vi "Check AI3 BAE7.vi"(0 "error in":errorcluster) -> (14 "error out":errorcluster, 16 "voltage out":dbl format="%#_13g")   [LabVIEW 2014]
doc: "Check AI3 BAE7\n\nThis returns the voltage inputted into AI3, which serves as the analog input receiving ~ 5 V through DC.\n\nBeverly Abadines\nPHY 350\nE7"
uses:
  <vilib>/DAQmx/read.llb/DAQmx Read.vi
  <vilib>/DAQmx/read.llb/DAQmx Read (Analog 1D DBL NChan 1Samp).vi
  <vilib>/DAQmx/miscellaneous.llb/DAQmx Fill In Error Info.vi
  <vilib>/DAQmx/create/channels.llb/DAQmx Create Channel (AI-Voltage-Basic).vi
  <vilib>/DAQmx/create/channels.llb/DAQmx Create Channel (TEDS-AI-Voltage-Basic).vi
panel:
  out "device out":tag="Dev1"
  in  "device in":tag="Dev1"
  in  "stop (T)":bool=TRUE
  in  "timeout (s)":dbl=10.0 format="%0.2f"
  out "task out":refnum<k21>
  # "Check AI3 BAE7"
  # "Beverly Abadines\nPhys 350\nE7"
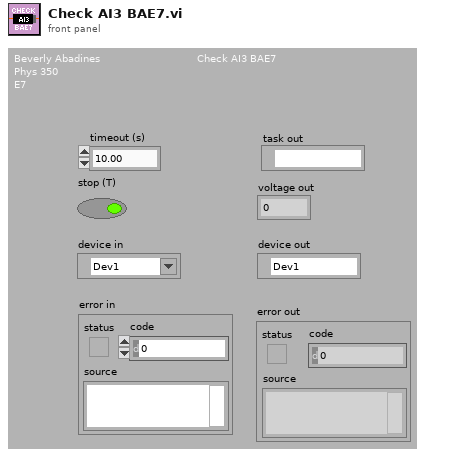
[diagram p1: front panel]
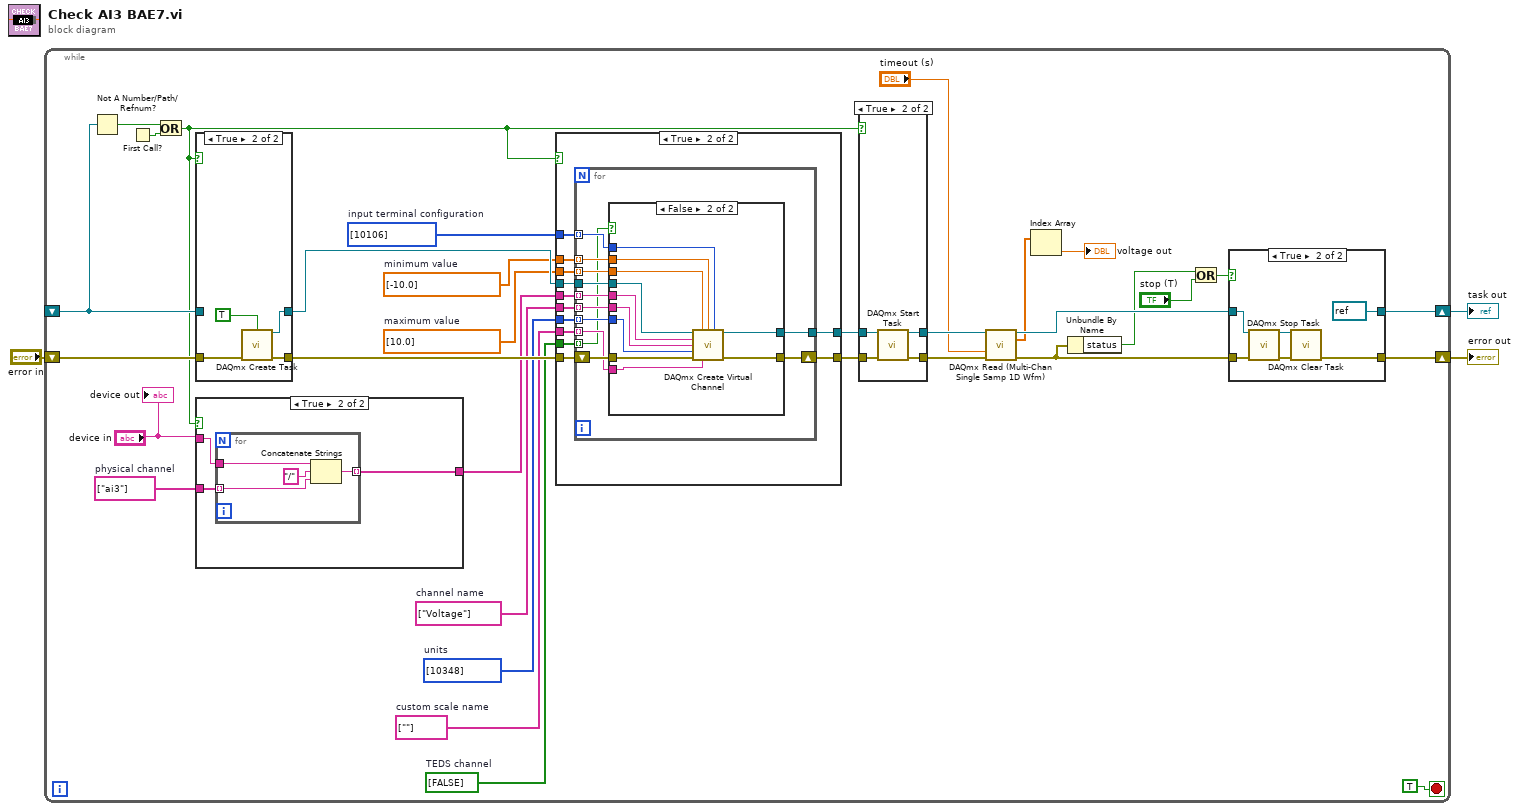
[diagram p0: block diagram]
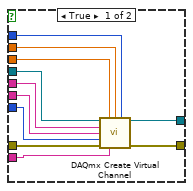
[diagram p5: hidden frame]
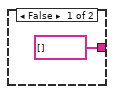
[diagram p6: hidden frame]
diagram:
  n1 = while {
    shift-right: [w12] -> w1
    shift-left: _ -> [w32]
    shift-right: [w10] -> w2
    shift-left: "error in" -> [w33]
    stop <- TRUE stop-if-true
    w19 = bool[] [FALSE]  # TEDS channel
    w20 = string[] [""]  # custom scale name
    w21 = i32[] [10348] items=["Volts"=10348, "From TEDS"=12516, "From Custom Scale"=10065]  # units
    w22 = string[] ["Voltage"]  # channel name
    w24 = dbl[] [10.0]  # maximum value
    w25 = dbl[] [-10.0]  # minimum value
    w26 = i32[] [10106] items=["default"=-1, "RSE"=10083, "NRSE"=10078, "Differential"=10106, "Pseudodifferential"=12529]  # input terminal configuration
    w29 = string[] ["ai3"]  # physical channel
    n2 = Not A Number/Path/Refnum?(number/path/refnum=w32) -> (NaN/Path/Refnum?=w31:bool)
    n3 = First Call?() -> (First Call?: T/F=w34:bool)
    n4 = Or(x=w31, y=w34) -> (x .or. y?=w18:bool)
    n5 = case shown="True" w18 {
      tunnel: [w107 w111] -> w28
      tunnel: w32 -> [w107 _]
      tunnel: [w106 w110] -> w27
      tunnel: w33 -> [w106 w108]
      frame False {
      }
      frame True {
        n6 = call <vilib>:"DAQmx Create Task.vi"("auto cleanup"=TRUE, "error in"=w108) -> ("task out"=w111:refnum<k21>, "error out"=w110:errorcluster)  [unwired: 12 in]
      }
    }
    n7 = case shown="True" w18 {
      tunnel: [string[] [] w101] -> w23
      tunnel: "device in" -> [_ w100]
      tunnel: w29 -> [_ w99]
      frame False {
      }
      frame True {
        n8 = for {
          tunnel: [w105] -> w101 mode=indexing
          tunnel: w100 -> [w104]
          tunnel: w99 -> [w102] mode=indexing
          n9 = Concatenate Strings(w104, "/" ("string"), w102) -> (w105:string)
        }
      }
    }
    n10 = case shown="True" w18 {
      tunnel: [w51 w61] -> w17
      tunnel: w28 -> [w51 w63]
      tunnel: [w50 w60] -> w16
      tunnel: w27 -> [w50 w62]
      tunnel: w26 -> [_ w59]
      tunnel: w25 -> [_ w58]
      tunnel: w24 -> [_ w57]
      tunnel: w23 -> [_ w56]
      tunnel: w22 -> [_ w55]
      tunnel: w21 -> [_ w54]
      tunnel: w20 -> [_ w53]
      tunnel: w19 -> [_ w52]
      frame False {
      }
      frame True {
        n11 = for {
          tunnel: w63 -> [w75]
          tunnel: [w73] -> w61
          tunnel: w59 -> [w71] mode=indexing
          tunnel: w58 -> [w70] mode=indexing
          tunnel: w57 -> [w69] mode=indexing
          tunnel: w56 -> [w68] mode=indexing
          tunnel: w55 -> [w67] mode=indexing
          tunnel: w54 -> [w66] mode=indexing
          tunnel: w53 -> [w65] mode=indexing
          shift-right: [w72] -> w60
          shift-left: w62 -> [w74]
          tunnel: w52 -> [w64] mode=indexing
          n12 = case shown="False" w64 {
            tunnel: w75 -> [w86 w97]
            tunnel: w74 -> [w85 w96]
            tunnel: [w84 w95] -> w73
            tunnel: [w83 w94] -> w72
            tunnel: w71 -> [w82 w93]
            tunnel: w70 -> [w81 w92]
            tunnel: w69 -> [w80 w91]
            tunnel: w68 -> [w79 w90]
            tunnel: w67 -> [w78 w89]
            tunnel: w66 -> [w77 w88]
            tunnel: w65 -> [w76 w87]
            frame True {
              n13 = call-poly <vilib>:"DAQmx Create Virtual Channel.vi"("task in"=w86, "maximum value"=w80, "minimum value"=w81, "input terminal configuration"=w82, "physical channels"=w79, "name to assign"=w78, "units"=w77, "error in"=w85, "custom scale name"=w76) -> ("task out"=w84:refnum<k21>, "error out"=w83:errorcluster)  [unwired: 5 in]
            }
            frame False {
              n14 = call-poly <vilib>:"DAQmx Create Virtual Channel.vi"("task in"=w97, "maximum value"=w91, "minimum value"=w92, "input terminal configuration"=w93, "physical channels"=w90, "name to assign"=w89, "units"=w88, "error in"=w96, "custom scale name"=w87) -> ("task out"=w95:refnum<k21>, "error out"=w94:errorcluster)  [unwired: 5 in]
            }
          }
        }
      }
    }
    n15 = case shown="True" w18 {
      tunnel: [w45 w48] -> w15
      tunnel: w17 -> [w45 w49]
      tunnel: [w44 w46] -> w14
      tunnel: w16 -> [w44 w47]
      frame False {
      }
      frame True {
        n16 = call <vilib>:"DAQmx Start Task.vi"("task/channels in"=w49, "error in"=w47) -> ("task out"=w48:refnum<k21>, "error out"=w46:errorcluster)  [unwired: 12 in]
      }
    }
    n17 = call-poly "DAQmx Read (Multi-Chan Single Samp 1D Wfm).vi"("task/channels in"=w15, "timeout"="timeout (s)", "error in"=w14) -> ("task out"=w11:refnum<k21>, "data"=w4:dbl[], "error out"=w9:errorcluster)  [unwired: 10 in]
    n18 = Index Array(array=w4) -> (element=→"voltage out":dbl)  [unwired: 1 in]
    n19 = Unbundle By Name(w9) -> ("status"=w8:bool)
    n20 = Or(x=w8, y="stop (T)") -> (x .or. y?=w6:bool)
    n21 = case shown="True" w6 {
      tunnel: [w37 refnum<k21> refnum ("task in")] -> w12
      tunnel: w11 -> [w37 w43]
      tunnel: [w36 w40] -> w10
      tunnel: w9 -> [w36 w42]
      frame False {
      }
      frame True {
        n22 = call <vilib>:"DAQmx Stop Task.vi"("task/channels in"=w43, "error in"=w42) -> ("task out"=w39:refnum<k21>, "error out"=w41:errorcluster)  [unwired: 12 in]
        n23 = call <vilib>:"DAQmx Clear Task.vi"("task in"=w39, "error in"=w41) -> ("error out"=w40:errorcluster)  [unwired: 13 in]
      }
    }
    "device out" <- "device in"
  }
  "error out" <- w2
  "task out" <- w1
